vi "Add Array Data Channels.vi"(8 "Error In":errorcluster, 10 "Array Elements":T2[](array[typedef]), 11 "Section Refnum In":T1 format="%.0x") -> (0 "Error Out":errorcluster, 3 "Channel Refnums":T1[](array[typedef]) format="%.0x")   [LabVIEW 2018, in "Instrument Addon Scripting API.lvlib"]
doc: "Adds channels under the Data Array section provided as reference input."
uses:
  Instrument Addon Scripting API.lvlib
  <vilib>/NI Veristand/Custom Device API/Custom Device Item Ref.ctl
  TypeDefs/Array Element.ctl
  <vilib>/NI Veristand/Custom Device API/Custom Device Channel.ctl
  <vilib>/NI Veristand/Custom Device API/Custom Device Channel Type.ctl
  Addon/Addon Shared/SubVIs/Constants.vi
  <vilib>/NI Veristand/Custom Device API/Custom Device API.lvlib
  Addon/Addon Shared/Instrument Addon Shared.lvlib
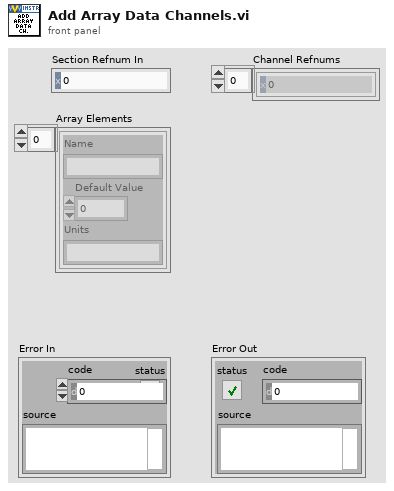
[diagram p1: front panel]
types:
  T1 = typedef "Custom Device API.lvlib/Custom Device Item Ref.ctl" = u64
  T2 = typedef "Instrument Addon Scripting API.lvlib/Array Element.ctl" = cluster{"Name":string, "Default Value":dbl, "Units":string}
  T3 = typedef "Custom Device API.lvlib/Custom Device Channel.ctl" = cluster{"Type":T4, "Units":string, "Default Value":dbl, "Faultable":bool, "Scalable":bool}
  T4 = typedef "Custom Device API.lvlib/Custom Device Channel Type.ctl" = enum16{"Input", "Output"}
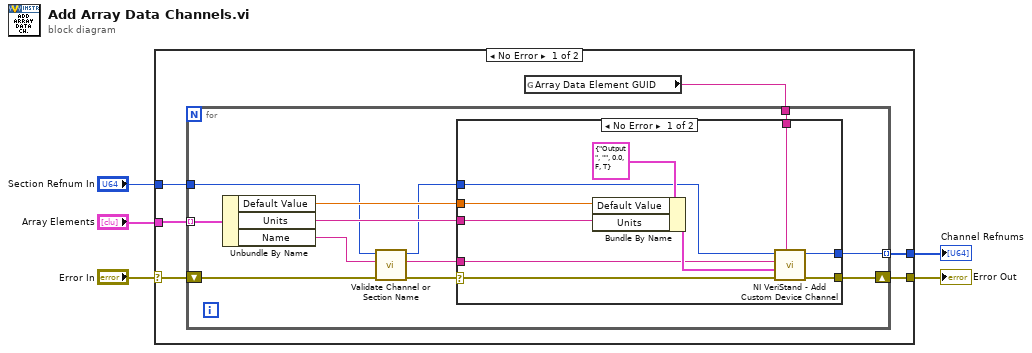
[diagram p0: block diagram]
diagram:
  n1 = case shown="No Error" "Error In" {
    selector: "Error In" -> [w8 w36]
    tunnel: [w11 w36] -> w5
    tunnel: "Section Refnum In" -> [w10 _]
    tunnel: "Array Elements" -> [w6 _]
    tunnel: [w7 _] -> w1
    frame No Error {
      n2 = global read "Constants.vi" "Array Data Element GUID"() -> (w9:string)
      n3 = for {
        shift-right: [w23] -> w11
        shift-left: w8 -> [w17]
        tunnel: w9 -> [w22]
        tunnel: w10 -> [w16]
        tunnel: w6 -> [w21] mode=indexing
        tunnel: [w18] -> w7 mode=indexing
        n4 = Unbundle By Name(w21) -> ("Default Value"=w20:dbl, "Units"=w19:string, "Name"=w13:string)
        n5 = call "Validate Channel or Section Name.vi"("error in (no error)"=w17, "Name In"=w13, "Refnum In"=w16) -> ("error out"=w12:errorcluster, "Name Out"=w14:string, "Refnum Out"=w15:T1)  [unwired: 6 in]
        n6 = case shown="No Error" w12 {
          selector: w12 -> [w24 w34]
          tunnel: [w33 w34] -> w23
          tunnel: w22 -> [w30 _]
          tunnel: w15 -> [w29 w35]
          tunnel: w20 -> [w28 _]
          tunnel: w19 -> [w27 _]
          tunnel: w14 -> [w26 _]
          tunnel: [w25 w35] -> w18
          frame No Error {
            n7 = Bundle By Name(cluster=T3 {"Type"=enum."Output", "Units"="", "Default Value"=0.0, "Faultable"=FALSE, "Scalable"=TRUE} ("Channel"), "Default Value"=w28, "Units"=w27) -> (w31:T3)
            n8 = call <vilib>:"NI VeriStand - Add Custom Device Channel.vi"("GUID (Default Channel)"=w30, "error in (no error)"=w24, "Channel"=w31, "Channel Name"=w26, "Parent Ref in"=w29) -> ("error out"=w33:errorcluster, "Parent Ref out"=w25:T1)  [unwired: 3 in, 2 out]
          }
          frame Error {
          }
        }
      }
    }
    frame Error {
    }
  }
  "Error Out" <- w5
  "Channel Refnums" <- w1
